vi "Overcome_Permissions.vi"(2 "append to file? (new file:F)":bool, 3 "path":path, 4 "refnum In":refnum<file>) -> (0 "error out":errorcluster, 1 "refnum Out":refnum<file>)   [LabVIEW 2010]
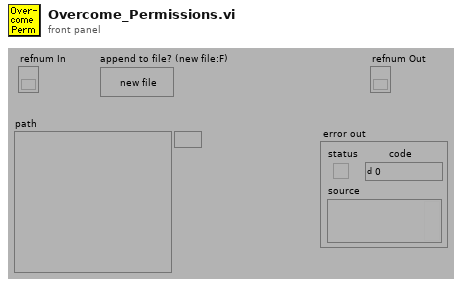
[diagram p1: front panel]
types:
  T1 = enum16{"open", "replace", "create", "open or create", "replace or create", "replace or create with confirmation"}
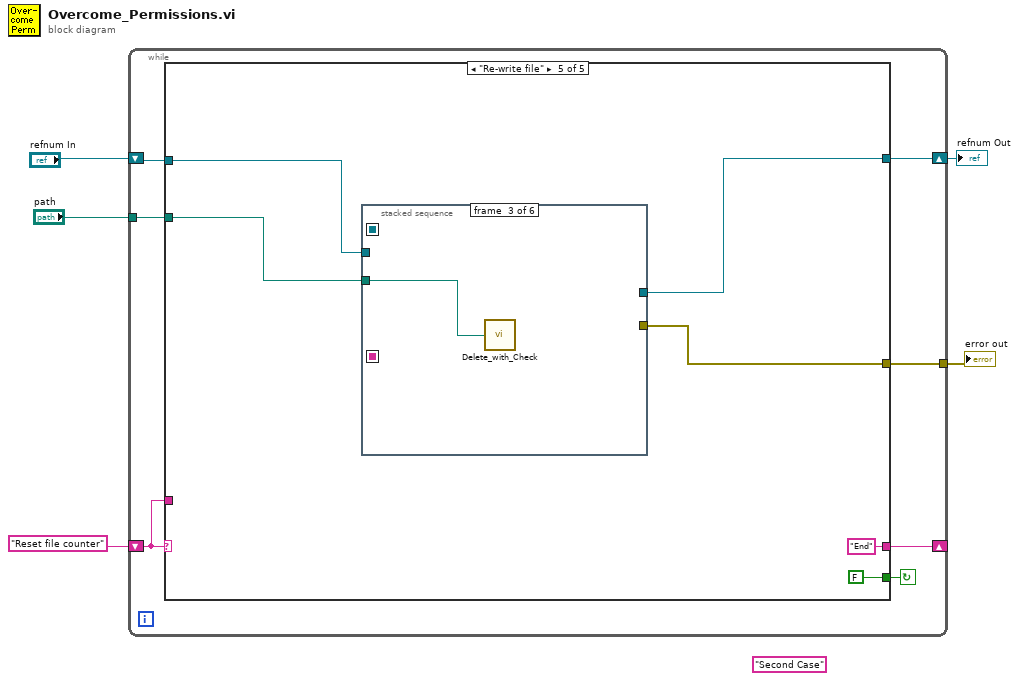
[diagram p0: block diagram]
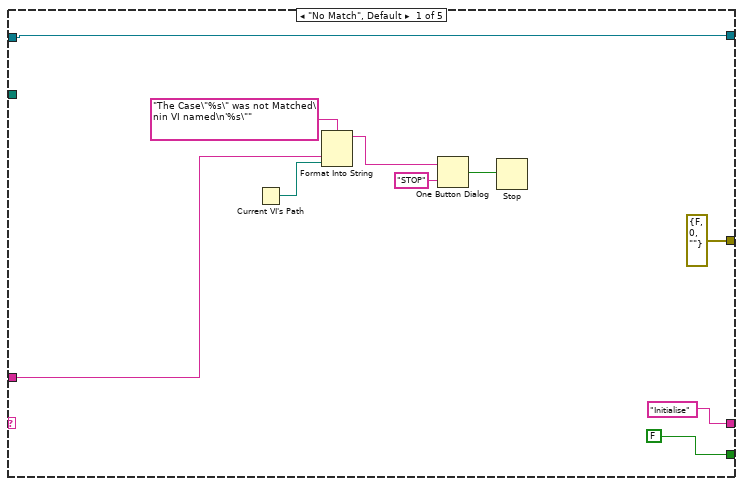
[diagram p2: hidden frame]
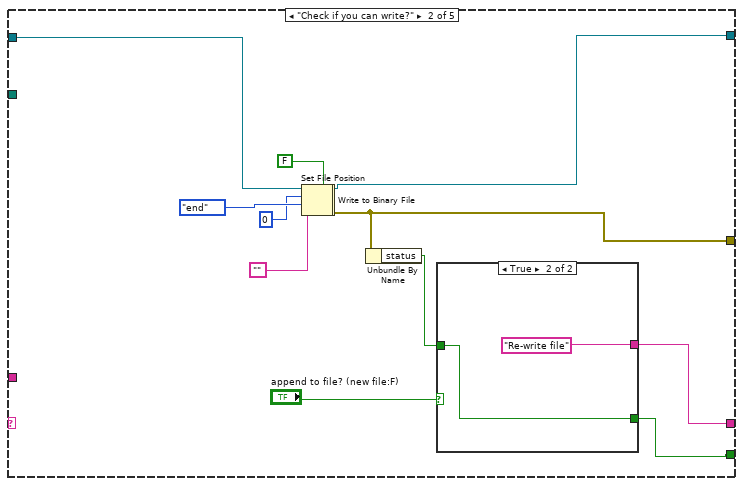
[diagram p3: hidden frame]
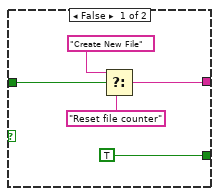
[diagram p4: hidden frame]
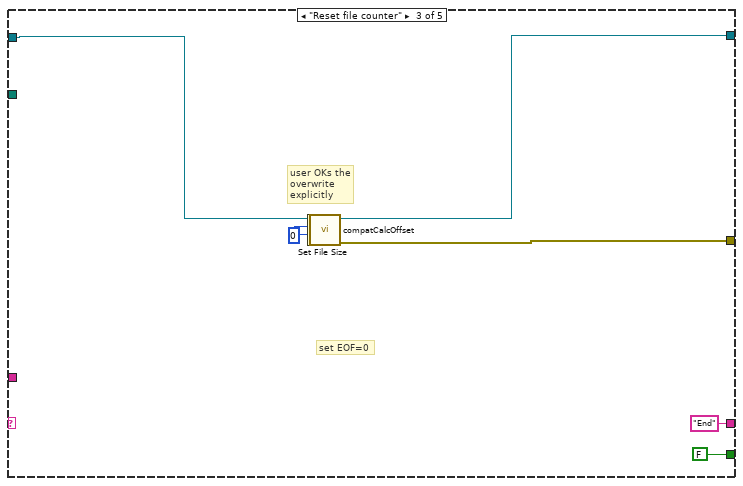
[diagram p5: hidden frame]
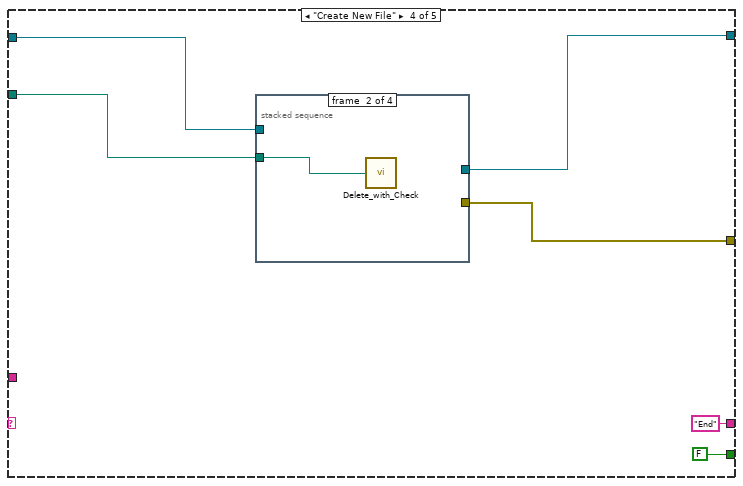
[diagram p6: hidden frame]
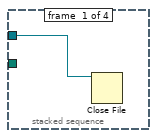
[diagram p7: hidden frame]
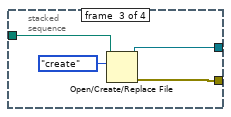
[diagram p8: hidden frame]
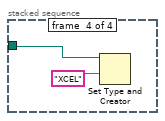
[diagram p9: hidden frame]
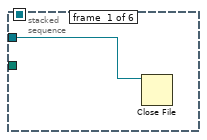
[diagram p10: hidden frame]
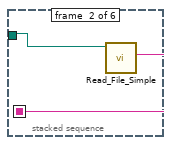
[diagram p11: hidden frame]
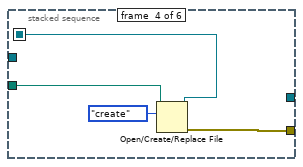
[diagram p12: hidden frame]
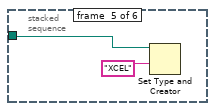
[diagram p13: hidden frame]
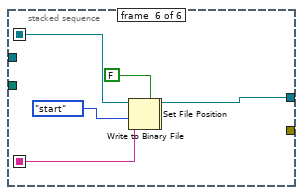
[diagram p14: hidden frame]
diagram:
  (unwired) "Second Case"
  n1 = while {
    shift-left: "Reset file counter" -> [w10]
    shift-right: [w11] -> _
    shift-right: [w8] -> w3
    shift-left: "refnum In" -> [w9]
    tunnel: "path" -> [w7]
    tunnel: [w6] -> w1
    stop <- w12 continue-if-true
    n2 = case shown="\"Re-write file\"" w10 {
      tunnel: [FALSE w27 FALSE FALSE FALSE] -> w12
      tunnel: ["Initialise" w26 "End" "End" "End"] -> w11
      tunnel: w10 -> [w17 _ _ _ _]
      tunnel: w9 -> [w14 w35 w50 w52 w66]
      tunnel: [w14 w30 w49 w54 w68] -> w8
      tunnel: w7 -> [_ _ _ w55 w69]
      tunnel: [errorcluster {"status"=FALSE, "code"=0, "source"=""} ("error out") w31 w46 w53 w67] -> w6
      frame "No Match", Default {
        n3 = Current VI's Path() -> (path=w16:path)
        n4 = Format Into String(format string="The Case\"%s\" was not Matched\nin VI named\n'%s\"" ("Format String"), w17, w16) -> (resulting string=w20:string)  [unwired: 2 in, 1 out]
        n5 = One Button Dialog(message=w20, button name ("OK")="STOP") -> (true=w18:bool)
        n6 = Stop(stop? (T)=w18) -> ()
      }
      frame "Check if you can write?" {
        n7 = Set File Position(offset (in bytes) (0)=0 ("pos offset (0)"), refnum=w35, from (0:start)=enum16{"start", "end", "current"}."end" ("pos mode (0:2)")) -> (refnum out=w25:refnum<file>, error out=w24:errorcluster)  [unwired: 1 in]
        n8 = Write to Binary File(file (use dialog)=w25, data="", error in=w24, 5:FALSE ("prepend array or string size? (T)")) -> (refnum out=w30:refnum<file>, error out=w31:errorcluster)  [unwired: 2 in, 1 out]
        n9 = Unbundle By Name(w31) -> ("status"=w32:bool)
        n10 = case shown="True" "append to file? (new file:F)" {
          tunnel: w32 -> [w40 w42]
          tunnel: [TRUE w42] -> w27
          tunnel: [w36 "Re-write file"] -> w26
          frame False {
            n11 = Select(t="Create New File", s=w40, f="Reset file counter") -> (s? t:f=w36:string)
          }
          frame True {
          }
        }
      }
      frame "Reset file counter" {
        w51 = 0
        # "set EOF=0"
        # "user OKs the overwrite explicitly"
        n12 = call <vilib>:"compatCalcOffset.vi"("pos offset (0)"=w51, "pos mode (0:1)"=w51, "refnum"=w50) -> ("error out"=w45:errorcluster, "offset"=w44:i32, "dup refnum"=w43:refnum<file>)  [unwired: 6 in]
        n13 = Set File Size(4:w45, 6:w44, 7:w43) -> (0:w46:errorcluster, 3:w49:refnum<file>)
      }
      frame "Create New File" {
        n14 = stacked-sequence {
          tunnel: [_ _ w63 _] -> w54
          tunnel: [_ _ w62 _] -> w53
          tunnel: w55 -> [_ w59 w61 w64]
          tunnel: w52 -> [w58 _ _ _]
          frame #0 {
            n15 = Close File(refnum=w58) -> ()  [unwired: 1 in, 2 out]
          }
          frame #1 {
            n16 = call "Delete_with_Check.vi"("FilePath"=w59) -> ()  [unwired: 1 out]
          }
          frame #2 {
            n17 = Open/Create/Replace File(file path (use dialog)=w61, operation (0:open)=T1."create") -> (refnum out=w63:refnum<file>, error out=w62:errorcluster)  [unwired: 4 in, 1 out]
          }
          frame #3 {
            n18 = Set Type and Creator(5:"XCEL", 7:w64) -> ()  [unwired: 2 in, 2 out]
          }
        }
      }
      frame "Re-write file" {
        n19 = stacked-sequence {
          seq-local: [_ w73 _ _ _ _] -> [_ _ _ _ _ w86]
          seq-local: [_ _ _ w77 _ _] -> [_ _ _ _ _ w88]
          tunnel: [_ _ _ _ _ w85] -> w68
          tunnel: [_ _ _ w79 _ _] -> w67
          tunnel: w69 -> [_ w74 w75 w78 w80 _]
          tunnel: w66 -> [w72 _ _ _ _ _]
          frame #0 {
            n20 = Close File(refnum=w72) -> ()  [unwired: 1 in, 2 out]
          }
          frame #1 {
            n21 = call "Read_File_Simple.vi"("Filename"=w74) -> ("string"=w73:string)  [unwired: 4 in, 5 out]
          }
          frame #2 {
            n22 = call "Delete_with_Check.vi"("FilePath"=w75) -> ()  [unwired: 1 out]
          }
          frame #3 {
            n23 = Open/Create/Replace File(file path (use dialog)=w78, operation (0:open)=T1."create") -> (refnum out=w77:refnum<file>, error out=w79:errorcluster)  [unwired: 4 in, 1 out]
          }
          frame #4 {
            n24 = Set Type and Creator(5:"XCEL", 7:w80) -> ()  [unwired: 2 in, 2 out]
          }
          frame #5 {
            n25 = Set File Position(refnum=w88, from (0:start)=enum16{"start", "end", "current"}."start" ("pos mode (0:2)")) -> (refnum out=w84:refnum<file>, error out=w83:errorcluster)  [unwired: 2 in]
            n26 = Write to Binary File(file (use dialog)=w84, data=w86, error in=w83, 5:FALSE ("prepend array or string size? (T)")) -> (refnum out=w85:refnum<file>)  [unwired: 2 in, 2 out]
          }
        }
      }
    }
  }
  "refnum Out" <- w3
  "error out" <- w1
